vi "set Modified Period.vi"(11 "Timer in":refnum<class "Timer.lvclass">) -> (3 "Timer out":refnum<class "Timer.lvclass">)   [LabVIEW 2015, in "Timer.lvclass"]
uses:
  Timer.lvclass
  Timer.lvclass/Timer.ctl
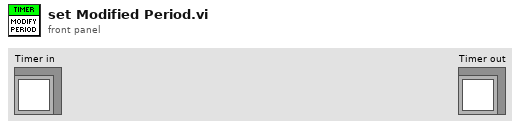
[diagram p1: front panel]
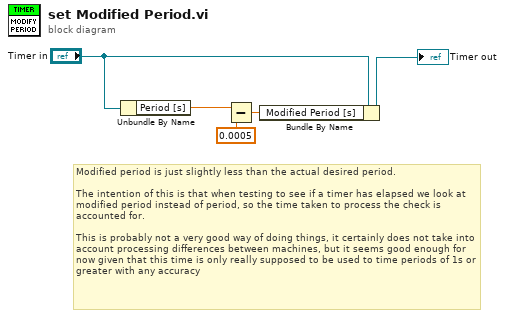
[diagram p0: block diagram]
diagram:
  # "Modified period is just slightly less than the actual desired period.\n\nThe intention of this is that when testing to see if a timer has elapsed we look at modified period instead of period, so the time taken to process the check is accounted for.\n\nThis is probably not a very good way of doing things, it certainly does not take into account processing differences between machines, but it seems good enough for now given that this time is only really supposed to be used to time periods of 1s or greater with any accuracy"
  n1 = Unbundle By Name("Timer in") -> ("Period [s]"=w4:dbl)
  n2 = Subtract(x=w4, y=0.0005) -> (x-y=w3:dbl)
  n3 = Bundle By Name(cluster="Timer in", "Modified Period [s]"=w3) -> (→"Timer out":refnum<class "Timer.lvclass">)
